vi "USB_control.vi"   [LabVIEW 2016]
uses:
  <vilib>/NXT/NXT Controls/ConnectionType.ctl
  <vilib>/NXT/LegoClasses/EV3/LED Pattern.ctl
  <vilib>/NXT/Block Support/NXT_OutputPort.ctl
  <vilib>/NXT/Dual Mode Library/Display/BrickLight.vi
  <vilib>/Utility/inputDevices.llb/keyboardAcquire.vi
  <vilib>/NXT/NXTIO Xnodes/NXTIONodeSubVIs/NXTStopMotors.vi
  <vilib>/NXT/NXTIO Xnodes/NXTIONodeSubVIs/NXTMoveMotors.vi
  <vilib>/NXT/Dual Mode Library/Sound/PlayE.vi
  <vilib>/NXT/Dual Mode Library/Sound/PlayC.vi
  <vilib>/NXT/Dual Mode Library/Sound/PlayG.vi
  <vilib>/NXT/Dual Mode Library/Waits/Wait_Num.vi
  <vilib>/Utility/inputDevices.llb/closeKeyboard.vi
  <vilib>/NXT/NXTIO Xnodes/AddressXNode/NXTIOAddress.xnode
  <vilib>/NXT/NXTIO Xnodes/NXTIOXNode/NXTIO.xnode
  <vilib>/NXT/Subs/LVHSConnector.ctl
  <vilib>/NXT/LegoClasses/BrickReference/BrickReference.lvclass
types:
  T1 = typedef "LED Pattern.ctl" = enum8{"None", "Green", "Red", "Orange", "Green Flash", "Red Flash", "Orange Flash", "Green Pulse", "Red Pulse", "Orange Pulse"}
  T2 = typedef "ConnectionType.ctl" = enum16{"Bluetooth", "USB", "WiFi"}
  T3 = typedef "LVHSConnector.ctl" = refnum<class "BrickReference.lvclass">
  T4 = enum16{"0", "1", "2", "3", "4", "5", "6", "7", "8", "9", "A", "B", "C", "D", "E", "F", "G", "H", "I", "J", "K", "L", "M", "N", "O", "P", "Q", "R", "S", "T", "U", "V", "W", "X", "Y", "Z", "F1", "F2", "F3", "F4", "F5", "F6", "F7", "F8", "F9", "F10", "F11", "F12", "F13", "F14", "F15", "ADD", "BACK", "BACKSLASH", "CAPITAL", "COMMA", "DECIMAL", "DELETE", "DIVIDE", "DOWN", "END", "EQUALS", "ESCAPE", "GRAVE (`)", "HOME", "INSERT", "LBRACKET", "LCONTROL", "LEFT", "L ALT", "LSHIFT", "LWIN", "MINUS", "MULTIPLY", "NEXT", "NUMLOCK", "NUMPAD_0", "NUMPAD_1", "NUMPAD_2", "NUMPAD_3", "NUMPAD_4", "NUMPAD_5", "NUMPAD_6", "NUMPAD_7", "NUMPAD_8", "NUMPAD_9", "PAUSE", "PERIOD", "PRIOR (PG UP)", "RBRACKET", "RCONTROL", "RETURN", "RIGHT", "R ALT", "RSHIFT", "RWIN", "SCROLL", "SEMICOLON", "SLASH", "SPACE", "SUBTRACT", "TAB", "UP", "ENTER (num pad)", "' (quote)"}
  T5 = typedef "NXT_OutputPort.ctl" = u8
  T6 = enum16{"0", "1", "2", "3", "4", "5", "6", "7", "8", "9", "A", "B", "C", "D", "E", "F", "G", "H", "I", "J", "K", "L", "M", "N", "O", "P", "Q", "R", "S", "T", "U", "V", "W", "X", "Y", "Z", "F1", "F2", "F3", "F4", "F5", "F6", "F7", "F8", "F9", "F10", "F11", "F12", "F13", "F14", "F15", "ADD", "BACK", "BACKSLASH", "CAPITAL", "COMMA", "DECIMAL", "DELETE", "DIVIDE", "DOWN", "END", "EQUALS", "ESCAPE", "GRAVE (`)", "HOME", "INSERT", "LBRACKET", "LCONTROL", "LEFT", "L ALT", "LSHIFT", "LWIN", "MINUS", "MULTIPLY", "NEXT", "NUMLOCK", "NUMPAD_0", "NUMPAD_1", "NUMPAD_2", "NUMPAD_3", "NUMPAD_4", "NUMPAD_5", "NUMPAD_6", "NUMPAD_7", "NUMPAD_8", "NUMPAD_9", "PAUSE", "PERIOD", "PRIOR (PG UP)", "RBRACKET", "RCONTROL", "RETURN", "RIGHT", "R ALT", "RSHIFT", "RWIN", "SCROLL", "SEMICOLON", "SLASH", "SPACE", "SUBTRACT", "TAB", "UP", "ENTER (num pad)", "' (quote)"}[]
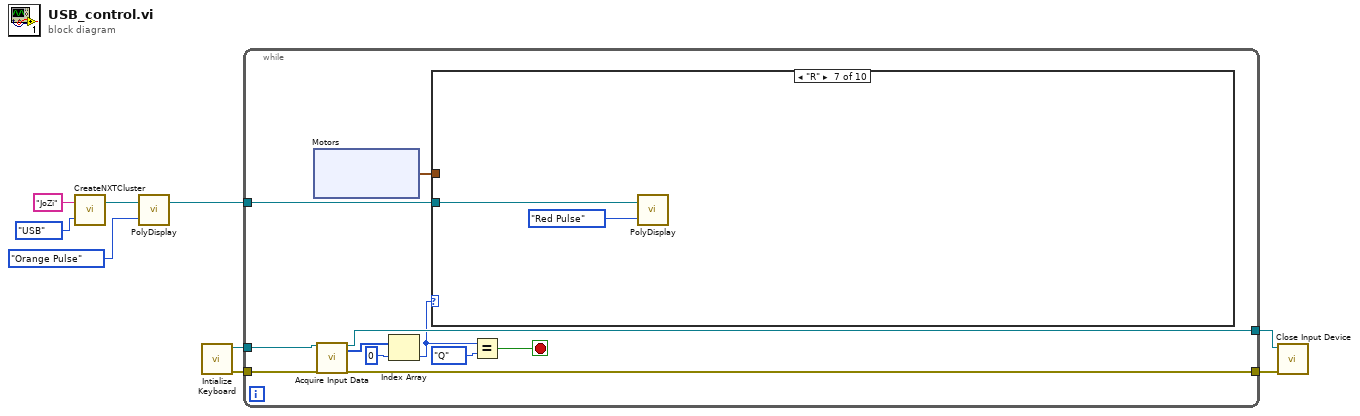
[diagram p0: block diagram]
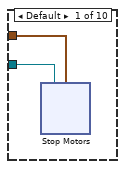
[diagram p2: hidden frame]
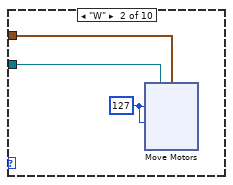
[diagram p3: hidden frame]
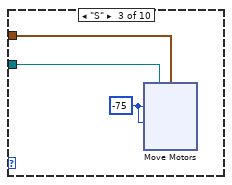
[diagram p4: hidden frame]
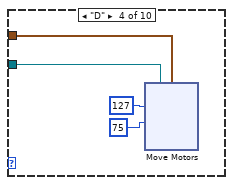
[diagram p5: hidden frame]
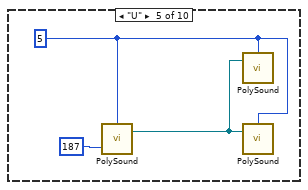
[diagram p6: hidden frame]
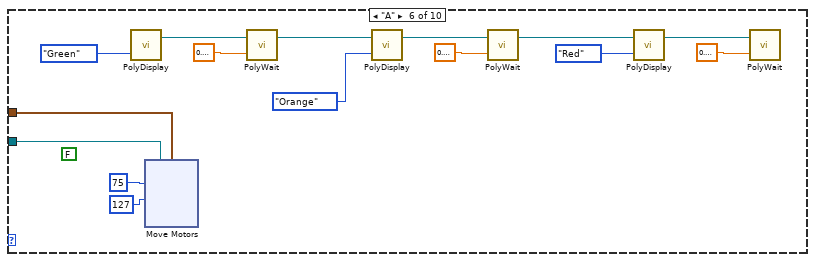
[diagram p7: hidden frame]
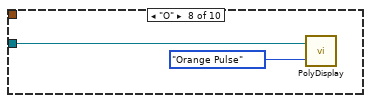
[diagram p8: hidden frame]
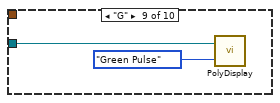
[diagram p9: hidden frame]
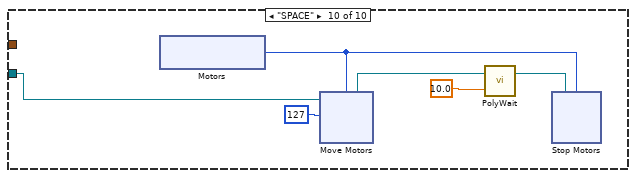
[diagram p10: hidden frame]
diagram:
  n1 = call <vilib>:"CreateNXTCluster.vi"("Connection Type"=ConnectionType."USB", "NXT/EV3 name"="JoZi") -> ("NXT/EV3"=w3:T3)  [unwired: 2 in]
  n2 = call-poly <vilib>:"PolyDisplay.vi"("Light Color"=LED_Pattern."Orange Pulse", "NXT/EV3"=w3) -> ("NXT/EV3"=w2:T3)  [unwired: 2 in]
  n3 = call <vilib>:"Intialize Keyboard.vi"() -> ("error out"=w5:errorcluster, "device ID"=w7:refnum<k1>)  [unwired: 10 in]
  n4 = while {
    tunnel: w7 -> [w20]
    tunnel: [w19] -> w6
    tunnel: w5 -> [w18]
    tunnel: [w17] -> w4
    tunnel: w2 -> [w13]
    stop <- w10 stop-if-true
    n5 = xnode "Motors"() -> ("Motor"=w14:cluster{"Port":T5, "Port":T5})
    n6 = call-poly <vilib>:"Acquire Input Data.vi"("device ID"=w20, "error in (no error)"=w18) -> ("device ID"=w19:refnum<k1>, "keys pressed"=w15:T6, "error out"=w17:errorcluster)  [unwired: 15 in]
    n7 = Index Array(array=w15, index=0) -> (element=w12:T4)
    n8 = case shown="\"R\"" w12 {
      tunnel: w14 -> [w23 w30 w42 w54 _ w78 _ _ _ _]
      tunnel: w13 -> [w22 w31 w41 w53 _ w80 w90 w92 w94 w100]
      frame Default {
        n9 = xnode "Stop Motors"("Motors"=w23, "NXT/EV3"=w22) -> ()  [unwired: 1 out]
      }
      frame "W" {
        w29 = i8 127 ("Power/Speed 1")
        n10 = xnode "Move Motors"("Power/Speed 2"=w29, "Power/Speed 1"=w29, "Motors"=w30, "NXT/EV3"=w31) -> ()  [unwired: 1 out]
      }
      frame "S" {
        w40 = i8 -75 ("Power/Speed 1")
        n11 = xnode "Move Motors"("Power/Speed 2"=w40, "Power/Speed 1"=w40, "Motors"=w42, "NXT/EV3"=w41) -> ()  [unwired: 1 out]
      }
      frame "D" {
        n12 = xnode "Move Motors"("Power/Speed 2"=i8 75, "Power/Speed 1"=i8 127, "Motors"=w54, "NXT/EV3"=w53) -> ()  [unwired: 1 out]
      }
      frame "U" {
        w63 = u16 5 ("Tone (440 Hz)")
        n13 = call-poly <vilib>:"PolySound.vi"("Duration (500 ms)"=u16 187, "Octave"=w63) -> ("NXT/EV3"=w64:T3)  [unwired: 2 in]
        n14 = call-poly <vilib>:"PolySound.vi"("NXT/EV3"=w64, "Octave"=w63) -> ()  [unwired: 2 in, 1 out]
        n15 = call-poly <vilib>:"PolySound.vi"("NXT/EV3"=w64, "Octave"=w63) -> ()  [unwired: 2 in, 1 out]
      }
      frame "A" {
        (unwired) FALSE
        n16 = call-poly <vilib>:"PolyDisplay.vi"("Light Color"=LED_Pattern."Green") -> ("NXT/EV3"=w73:T3)  [unwired: 3 in]
        n17 = xnode "Move Motors"("Power/Speed 2"=i8 127, "Power/Speed 1"=i8 75, "Motors"=w78, "NXT/EV3"=w80) -> ()  [unwired: 1 out]
        n18 = call-poly <vilib>:"PolyWait.vi"("Time (1 sec)"=sgl 0.2, "NXT/EV3"=w73) -> ("NXT/EV3"=w72:T3)  [unwired: 2 in]
        n19 = call-poly <vilib>:"PolyDisplay.vi"("Light Color"=LED_Pattern."Orange", "NXT/EV3"=w72) -> ("NXT/EV3"=w70:T3)  [unwired: 2 in]
        n20 = call-poly <vilib>:"PolyWait.vi"("Time (1 sec)"=sgl 0.2, "NXT/EV3"=w70) -> ("NXT/EV3"=w69:T3)  [unwired: 2 in]
        n21 = call-poly <vilib>:"PolyDisplay.vi"("Light Color"=LED_Pattern."Red", "NXT/EV3"=w69) -> ("NXT/EV3"=w67:T3)  [unwired: 2 in]
        n22 = call-poly <vilib>:"PolyWait.vi"("Time (1 sec)"=sgl 0.2, "NXT/EV3"=w67) -> ()  [unwired: 2 in, 1 out]
      }
      frame "R" {
        n23 = call-poly <vilib>:"PolyDisplay.vi"("Light Color"=LED_Pattern."Red Pulse", "NXT/EV3"=w90) -> ()  [unwired: 2 in, 1 out]
      }
      frame "O" {
        n24 = call-poly <vilib>:"PolyDisplay.vi"("Light Color"=LED_Pattern."Orange Pulse", "NXT/EV3"=w92) -> ()  [unwired: 2 in, 1 out]
      }
      frame "G" {
        n25 = call-poly <vilib>:"PolyDisplay.vi"("Light Color"=LED_Pattern."Green Pulse", "NXT/EV3"=w94) -> ()  [unwired: 2 in, 1 out]
      }
      frame "SPACE" {
        n26 = xnode "Motors"() -> ("Motor"=w95:T5)
        n27 = xnode "Move Motors"("Power/Speed 1"=i8 127, "Motors"=w95, "NXT/EV3"=w100) -> ("NXT/EV3"=w98:T3)
        n28 = call-poly <vilib>:"PolyWait.vi"("Time (1 sec)"=sgl 10.0, "NXT/EV3"=w98) -> ("NXT/EV3"=w96:T3)  [unwired: 2 in]
        n29 = xnode "Stop Motors"("Motors"=w95, "NXT/EV3"=w96) -> ()  [unwired: 1 out]
      }
    }
    n30 = Equal?(x=w12, y=T4."Q") -> (x = y?=w10:bool)
  }
  n31 = call-poly <vilib>:"Close Input Device.vi"("error in (no error)"=w4, "device ID"=w6) -> ()  [unwired: 8 in, 1 out]
